vi "[HOST] UTILITIES Calculate Spectrum.vi"(7 "Samples per Port":u32, 10 "Sample rate (Hz)":dbl format="%#_6p", 11 "Data":u64[](array[numeric])) -> (2 "Array":waveform(cdb)[](array[waveform]), 3 "Spectrum":cluster{"f0":dbl, "df":dbl, "magnitude":dbl[]}[](array[cluster]))   [LabVIEW 2016]
uses:
  <vilib>/measure/maspectr.llb/FFT Power Spectrum and PSD for 1 Chan (CDB).vi
  <vilib>/measure/NI_MAPro.lvlib
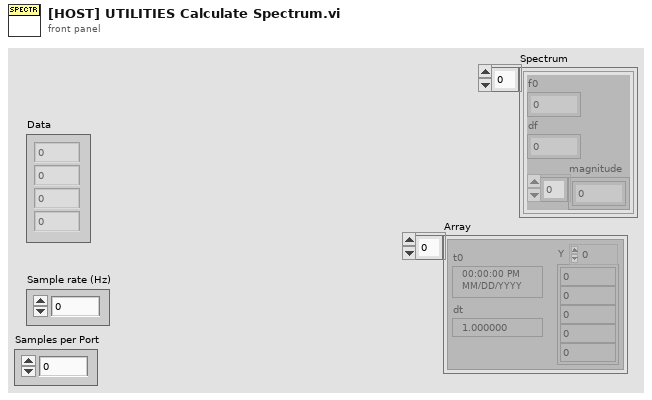
[diagram p1: front panel]
types:
  T1 = cluster{"averaging mode":enum16{"No averaging", "Vector averaging", "RMS averaging", "Peak hold"}, "weighting mode":enum16{"Linear", "Exponential"}, "number of averages":u32}
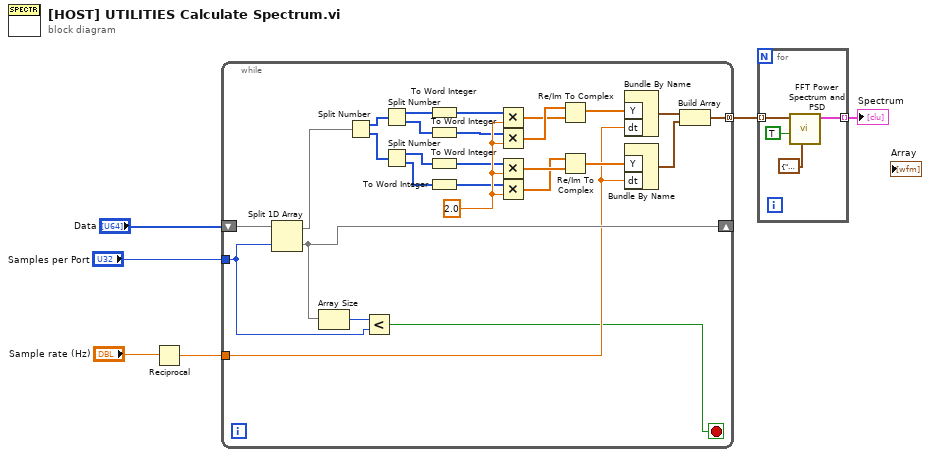
[diagram p0: block diagram]
diagram:
  n1 = Reciprocal(x="Sample rate (Hz)") -> (1/x=w3:dbl)
  n2 = while {
    tunnel: "Samples per Port" -> [w30]
    shift-right: [w32] -> _
    shift-left: "Data" -> [w33]
    tunnel: w3 -> [w11]
    tunnel: [w8] -> w2 mode=concatenating
    stop <- w7 stop-if-true
    w29 = 2.0
    n3 = Split 1D Array(array=w33, index=w30) -> (first subarray=w18:u64[], second subarray=w32:u64[])
    n4 = Array Size(array=w32) -> (size(s)=w31:i32)
    n5 = Split Number(x=w18) -> (hi(x)=w20:u32[], lo(x)=w19:u32[])
    n6 = Less?(x=w31, y=w30) -> (x < y?=w7:bool)
    n7 = Split Number(x=w20) -> (hi(x)=w21:u16[], lo(x)=w22:u16[])
    n8 = Split Number(x=w19) -> (hi(x)=w24:u16[], lo(x)=w26:u16[])
    n9 = To Word Integer(number=w21) -> (16bit integer=w23:i16[])
    n10 = To Word Integer(number=w22) -> (16bit integer=w25:i16[])
    n11 = To Word Integer(number=w24) -> (16bit integer=w27:i16[])
    n12 = To Word Integer(number=w26) -> (16bit integer=w28:i16[])
    n13 = Multiply(x=w23, y=w29) -> (x*y=w16:dbl[])
    n14 = Multiply(x=w25, y=w29) -> (x*y=w17:dbl[])
    n15 = Multiply(x=w27, y=w29) -> (x*y=w15:dbl[])
    n16 = Multiply(x=w28, y=w29) -> (x*y=w14:dbl[])
    n17 = Re/Im To Complex(1:w16, 2:w17) -> (0:w13:cdb[])
    n18 = Re/Im To Complex(1:w15, 2:w14) -> (0:w12:cdb[])
    n19 = Bundle By Name("Y"=w13, "dt"=w11) -> (w10:waveform(cdb))  [unwired: 1 in]
    n20 = Bundle By Name("Y"=w12, "dt"=w11) -> (w9:waveform(cdb))  [unwired: 1 in]
    n21 = Build Array(w10, w9) -> (w8:waveform(cdb)[])
  }
  n22 = for {
    tunnel: w2 -> [w37] mode=indexing
    tunnel: [w35] -> w1 mode=indexing
    n23 = call-poly <vilib>:"FFT Power Spectrum and PSD.vi"("averaging parameters"=T1 {"averaging mode"=enum."No averaging", "weighting mode"=enum."Exponential", "number of averages"=1}, "dB On (F)"=TRUE, "time signal"=w37) -> ("Power Spectrum / PSD"=w35:cluster{"f0":dbl, "df":dbl, "magnitude":dbl[]})  [unwired: 5 in, 3 out]
  }
  "Spectrum" <- w1
